vi "Generate short CSV Report.vi"(0 "Serial Number":string, 1 "Date":string, 2 "Time":string, 3 "Retest":string, 4 "Lower Limits":dbl, 5 "Measurment values":dbl, 6 "Fixture":string, 7 "Upper Limits":dbl, 8 "Variant":string, 9 "Status":string, 10 "Project":string, 11 "Overall status":string, 12 "Work Order":string, 13 "Test Names":string) -> (19 "error out":errorcluster)   [LabVIEW 2020, in "CSV Report.lvlib"]
uses:
  CSV Report.lvlib
  <vilib>/Utility/file.llb/Write Delimited Spreadsheet (string).vi
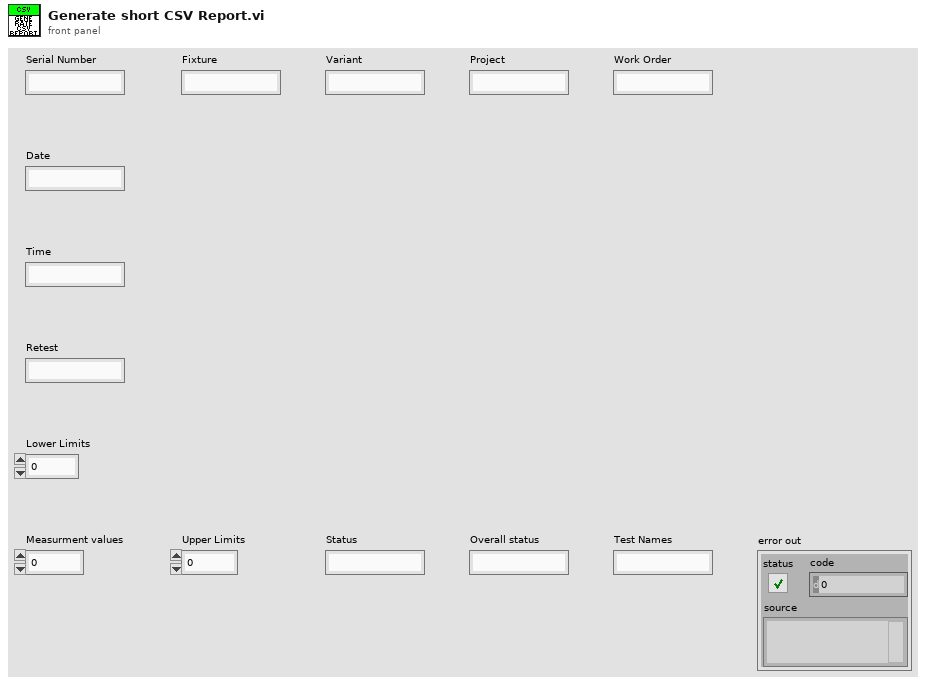
[diagram p1: front panel]
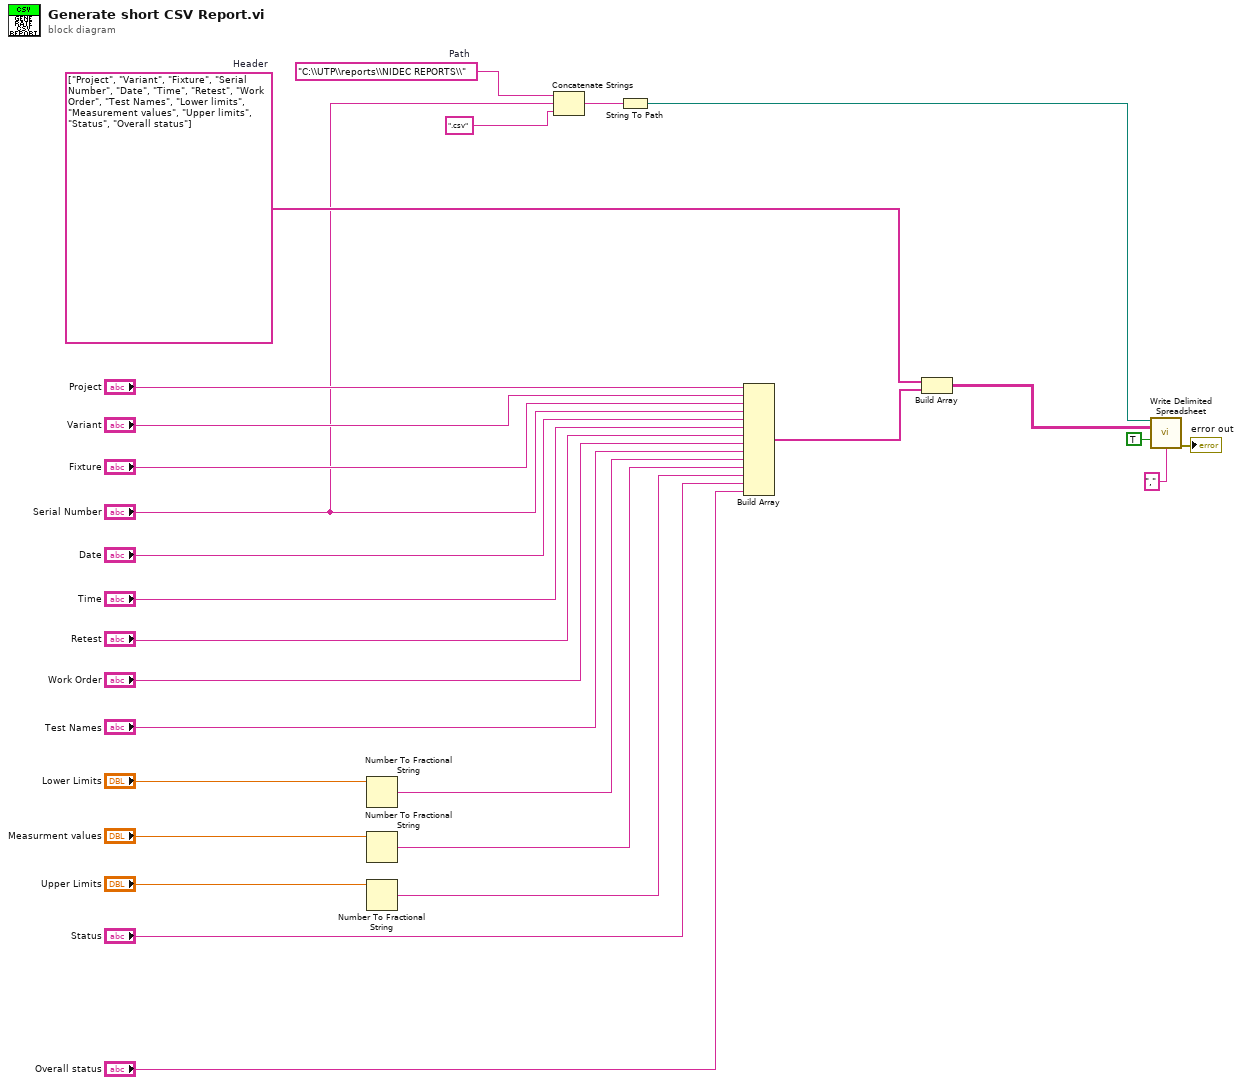
[diagram p0: block diagram]
diagram:
  w22 = "C:\\UTP\\reports\\NIDEC REPORTS\\"  # Path
  w25 = string[] ["Project", "Variant", "Fixture", "Serial Number", "Date", "Time", "Retest", "Work Order", "Test Names", "Lower limits", "Measurement values", "Upper limits", "Status", "Overall status"]  # Header
  n1 = Number To Fractional String(number="Lower Limits") -> (F-format string=w6:string)  [unwired: 3 in]
  n2 = Number To Fractional String(number="Measurment values") -> (F-format string=w3:string)  [unwired: 3 in]
  n3 = Number To Fractional String(number="Upper Limits") -> (F-format string=w2:string)  [unwired: 3 in]
  n4 = Concatenate Strings(w22, "Serial Number", ".csv" ("string")) -> (w21:string)
  n5 = String To Path(string=w21) -> (path=w20:path)
  n6 = Build Array("Project", "Variant", "Fixture", "Serial Number", "Date", "Time", "Retest", "Work Order", "Test Names", w6, w3, w2, "Status", "Overall status") -> (w24:string[])
  n7 = Build Array(w25, w24) -> (w23:string[][])
  n8 = call-poly <vilib>:"Write Delimited Spreadsheet.vi"("file path (dialog if empty)"=w20, "2D data"=w23, "append to file? (new file:F)"=TRUE, "delimiter (\\t)"="," ("delimiter (\\t)")) -> ("error out"=→"error out":errorcluster)  [unwired: 10 in, 1 out]
